vi "sub_file-path2.vi"(7 "cmd":T1, 8 "error in":errorcluster caption="error out") -> (0 "error out":errorcluster, 1 "Raw log file path":path, 3 "result path":path)   [LabVIEW 2016]
uses:
  ctl/file_path-cmd.ctl
  Global.vi
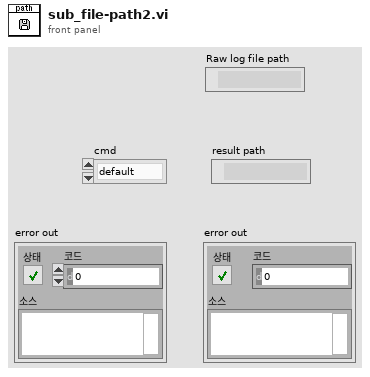
[diagram p1: front panel]
types:
  T1 = typedef "file_path-cmd.ctl" = enum16{"default", "write"}
  T2 = enum16{"open", "replace", "create", "open or create", "replace or create", "replace or create with confirmation"}
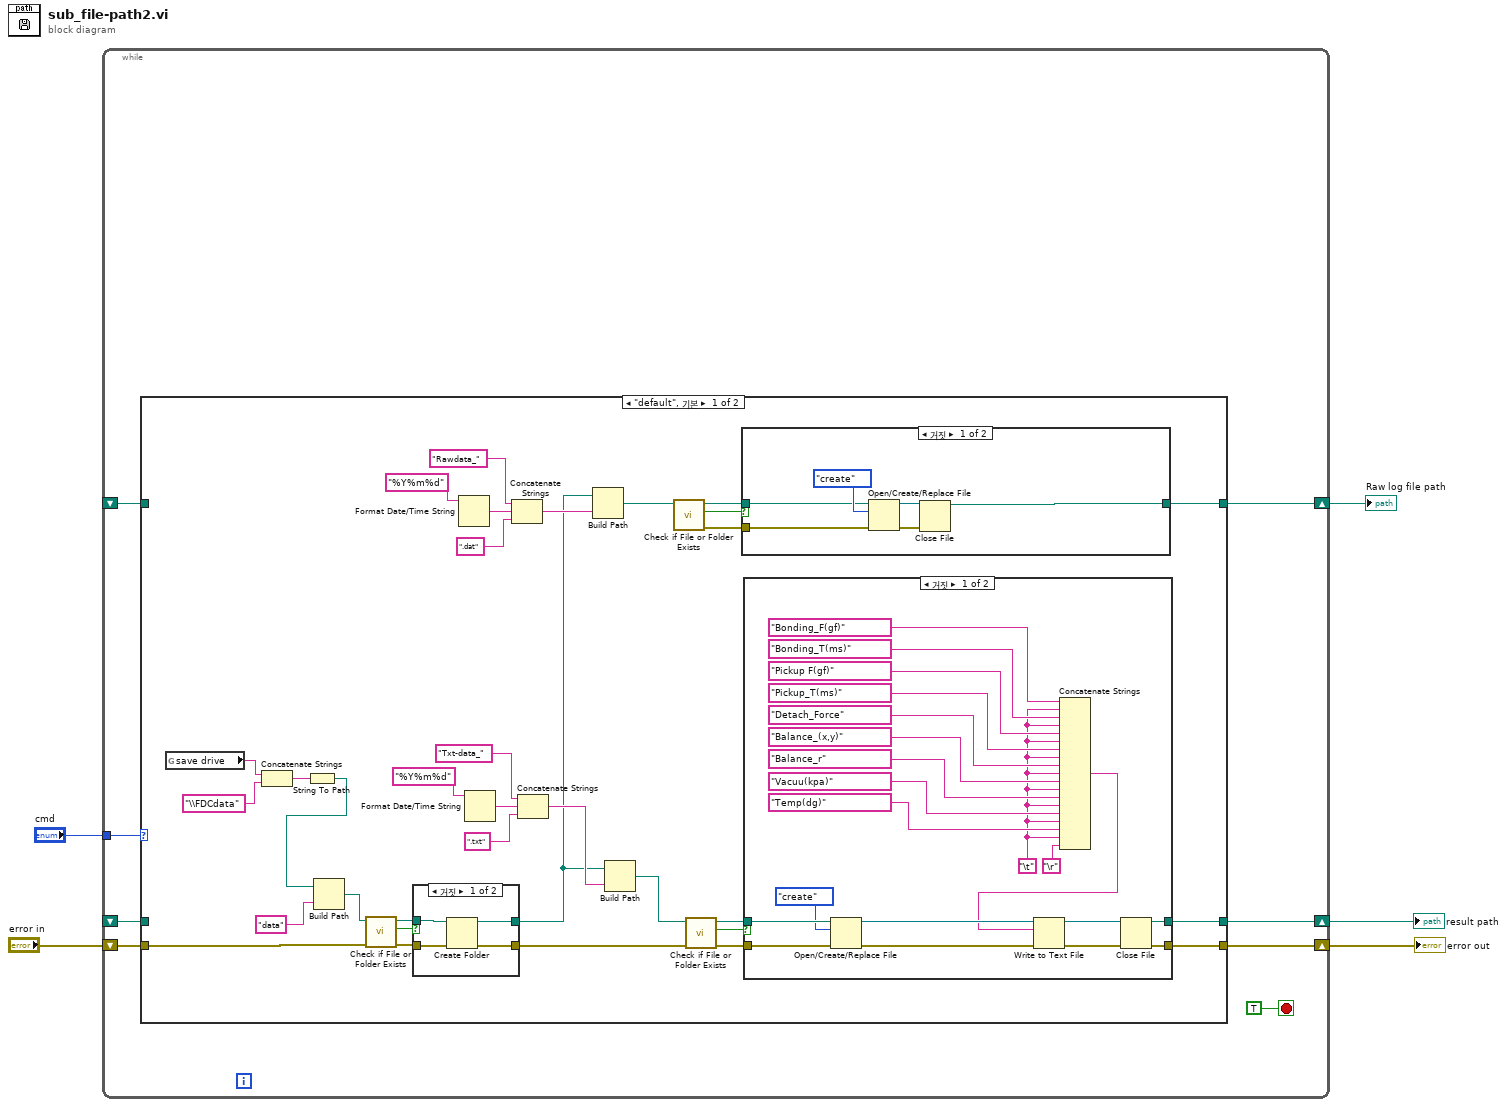
[diagram p0: block diagram]
diagram:
  n1 = while {
    tunnel: "cmd" -> [w12]
    shift-right: [w9] -> w4
    shift-left: _ -> [w8]
    shift-right: [w10] -> w3
    shift-left: "error in" -> [w11]
    shift-right: [w7] -> w2
    shift-left: _ -> [w6]
    stop <- TRUE stop-if-true
    n2 = case shown="\"default\", 기본" w12 {
      tunnel: w11 -> [w34 w85]
      tunnel: [w33 w85] -> w10
      tunnel: [w32 w84] -> w9
      tunnel: w8 -> [_ w84]
      tunnel: [w27 w83] -> w7
      tunnel: w6 -> [_ w83]
      frame "default", Default {
        n3 = global read "Global.vi" "save drive"() -> (w16:string)
        n4 = Concatenate Strings(w16, "\\FDCdata" ("이름 또는 상대 경로")) -> (w15:string)
        n5 = String To Path(string=w15) -> (path=w14:path)
        n6 = Build Path(base path=w14, name or relative path="data" ("이름 또는 상대 경로")) -> (appended path=w43:path)
        n7 = call <vilib>:"Check if File or Folder Exists.vi"("error in (no error)"=w34, "path"=w43) -> ("error out"=w46:errorcluster, "file or folder exists?"=w45:bool, "dup path"=w44:path)  [unwired: 7 in]
        n8 = case shown="거짓" w45 {
          tunnel: w44 -> [w80 w82]
          tunnel: w46 -> [w79 w81]
          tunnel: [w78 w82] -> w19
          tunnel: [w77 w81] -> w35
          frame False {
            n9 = Create Folder(path (use dialog)=w80, error in=w79) -> (created path=w78:path, error out=w77:errorcluster)  [unwired: 1 in, 1 out]
          }
          frame True {
          }
        }
        n10 = Format Date/Time String(time format string (%c)="%Y%m%d" ("시간 포맷 문자열 (%c)")) -> (date/time string=w23:string)  [unwired: 2 in]
        n11 = Format Date/Time String(time format string (%c)="%Y%m%d" ("시간 포맷 문자열 (%c)")) -> (date/time string=w37:string)  [unwired: 2 in]
        n12 = Concatenate Strings("Rawdata_" ("이름 또는 상대 경로"), w23, ".dat" ("문자열")) -> (w20:string)
        n13 = Concatenate Strings("Txt-data_" ("이름 또는 상대 경로"), w37, ".txt" ("문자열")) -> (w40:string)
        n14 = Build Path(base path=w19, name or relative path=w20) -> (appended path=w28:path)
        n15 = Build Path(base path=w19, name or relative path=w40) -> (appended path=w39:path)
        n16 = call <vilib>:"Check if File or Folder Exists.vi"("path"=w28) -> ("error out"=w25:errorcluster, "file or folder exists?"=w26:bool, "dup path"=w18:path)  [unwired: 8 in]
        n17 = call <vilib>:"Check if File or Folder Exists.vi"("error in (no error)"=w35, "path"=w39) -> ("error out"=w31:errorcluster, "file or folder exists?"=w30:bool, "dup path"=w29:path)  [unwired: 7 in]
        n18 = case shown="거짓" w26 {
          tunnel: [w49 w53] -> w27
          tunnel: w25 -> [w48 _]
          tunnel: w18 -> [w47 w53]
          frame False {
            n19 = Open/Create/Replace File(file path (use dialog)=w47, error in=w48, operation (0:open)=T2."create" ("동작(0:open)")) -> (refnum out=w50:refnum<file>, error out=w51:errorcluster)  [unwired: 3 in, 1 out]
            n20 = Close File(refnum=w50, error in=w51) -> (path=w49:path)  [unwired: 1 out]
          }
          frame True {
          }
        }
        n21 = case shown="거짓" w30 {
          tunnel: w29 -> [w74 w75]
          tunnel: w31 -> [w73 w76]
          tunnel: [w67 w76] -> w33
          tunnel: [w61 w75] -> w32
          frame False {
            w54 = "\t"
            n22 = Open/Create/Replace File(file path (use dialog)=w74, error in=w73, operation (0:open)=T2."create" ("동작(0:open)")) -> (refnum out=w70:refnum<file>, error out=w71:errorcluster)  [unwired: 3 in, 1 out]
            n23 = Concatenate Strings("Bonding_F(gf)", w54, "Bonding_T(ms)", w54, "Pickup F(gf)", w54, "Pickup_T(ms)", w54, "Detach_Force", w54, "Balance_(x,y)", w54, "Balance_r", w54, "Vacuu(kpa)", w54, "Temp(dg)", w54, "\r") -> (w62:string)
            n24 = Write to Text File(file (use dialog)=w70, text=w62, error in=w71) -> (refnum out=w69:refnum<file>, error out=w68:errorcluster)  [unwired: 1 in, 1 out]
            n25 = Close File(refnum=w69, error in=w68) -> (path=w61:path, error out=w67:errorcluster)
          }
          frame True {
          }
        }
      }
      frame "write" {
      }
    }
  }
  "result path" <- w4
  "error out" <- w3
  "Raw log file path" <- w2
